vi "Close Report File.vi"(8 "error in (no error)":errorcluster, 11 "Text Report In":refnum<class "Text Report.lvclass">) -> (0 "error out":errorcluster, 2 "Report Path":path)   [LabVIEW 2020, in "Text Report.lvclass"]
uses:
  Text Report.lvclass
  Text Report.lvclass/Text Report.ctl
  <vilib>/Platform/browser.llb/Open URL in Default Browser (path).vi
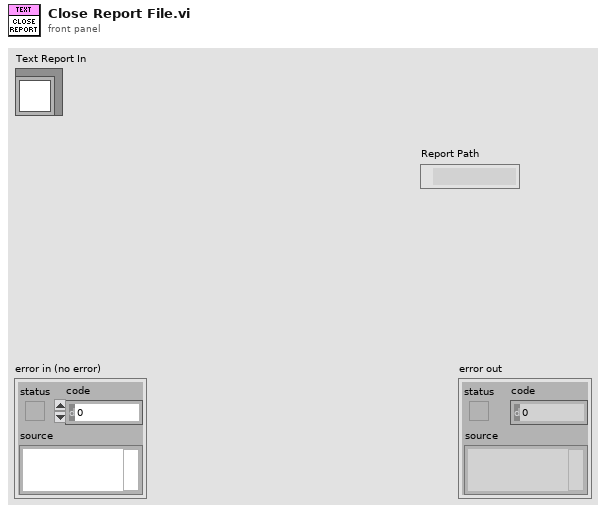
[diagram p1: front panel]
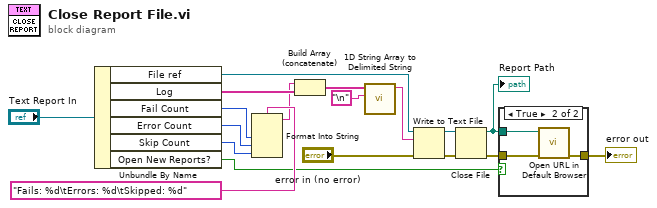
[diagram p0: block diagram]
diagram:
  n1 = Unbundle By Name("Text Report In") -> ("File ref"=w15:refnum<file>, "Log"=w12:string[], "Fail Count"=w8:i32, "Error Count"=w7:i32, "Skip Count"=w6:i32, "Open New Reports?"=w4:bool)
  n2 = Format Into String(format string="Fails: %d\tErrors: %d\tSkipped: %d", w8, w7, w6) -> (resulting string=w9:string)  [unwired: 2 in, 1 out]
  n3 = Build Array (concatenate)(w9, w12) -> (w5:string[])
  n4 = call <vilib>:"1D String Array to Delimited String.vi"("delimiter"="\n", "string array"=w5) -> ("delimited string"=w11:string)  [unwired: 9 in]
  n5 = Write to Text File(file (use dialog)=w15, text=w11, error in="error in (no error)") -> (refnum out=w14:refnum<file>, error out=w16:errorcluster)  [unwired: 1 in, 1 out]
  n6 = Close File(refnum=w14, error in=w16) -> (path=w3:path, error out=w1:errorcluster)
  "Report Path" <- w3
  n7 = case shown="True" w4 {
    tunnel: w3 -> [_ w20]
    tunnel: w1 -> [w19 w22]
    tunnel: [w19 w21] -> w2
    frame False {
    }
    frame True {
      n8 = call-poly <vilib>:"Open URL in Default Browser.vi"("error in (no error)"=w22, "path"=w20) -> ("error out"=w21:errorcluster)  [unwired: 4 in, 1 out]
    }
  }
  "error out" <- w2
